vi "Prepare Elves - Unique Movement Order.vi"(1 "Movement Proposal Rules":T2(array[cluster]), 2 "Elves' Positions":bool[][](array[boolean])) -> (0 "Elves with Unique Movement Order":T3(c390))   [LabVIEW 2020, in "AoC 2022.lvlib"]
uses:
  AoC 2022.lvlib
  Day 15 - Beacon Exclusion Zone/private/Location.ctl
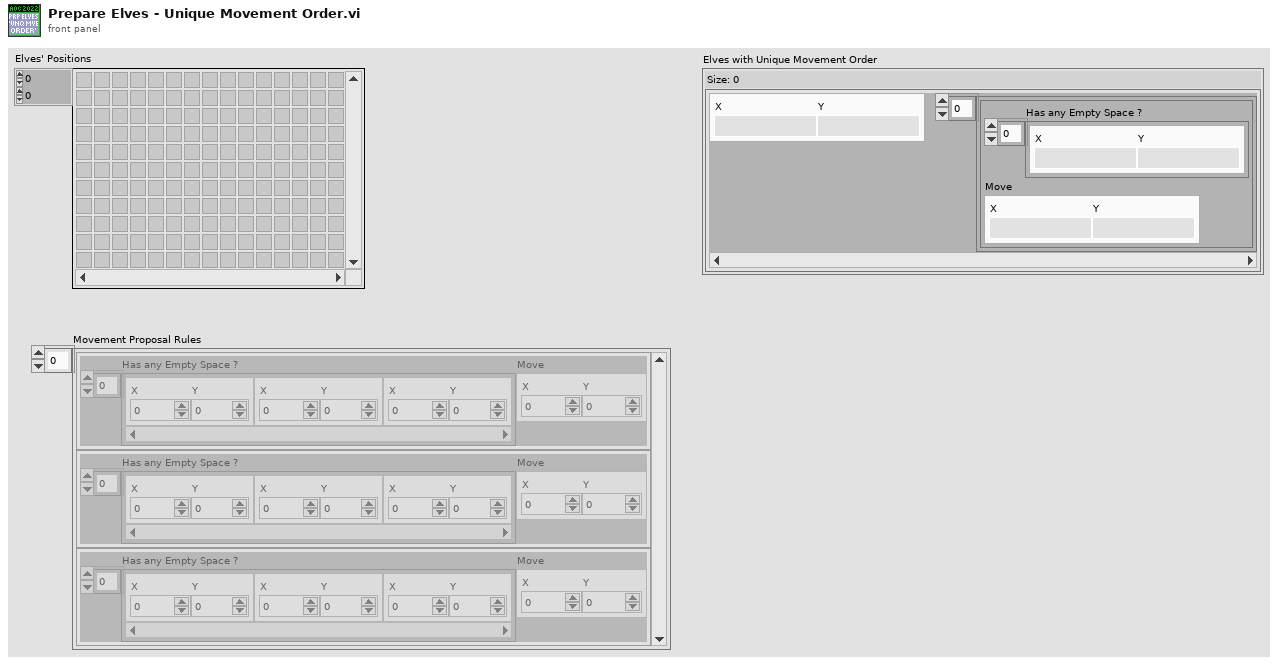
[diagram p1: front panel]
types:
  T1 = typedef "AoC 2022.lvlib/Location.ctl" = cluster{"X":i32, "Y":i32}
  T2 = cluster{"Has any Empty Space ?":T1[], "Move":T1}[]
  T3 = map{T1, cluster{"Has any Empty Space ?":T1[], "Move":T1}[]}
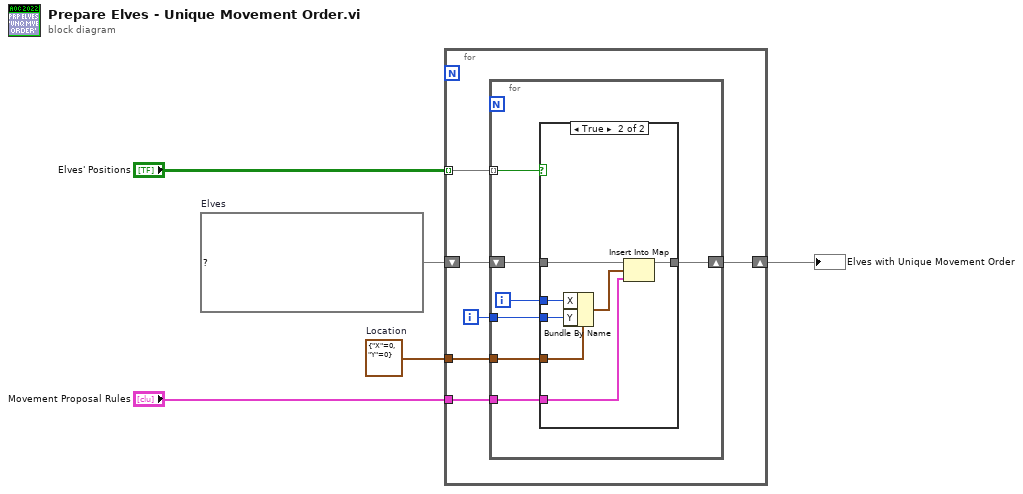
[diagram p0: block diagram]
diagram:
  w4 = T3 {}  # Elves
  w2 = T1 {"X"=0, "Y"=0}  # Location
  n1 = for {
    tunnel: "Elves' Positions" -> [w9] mode=indexing
    shift-right: [w11] -> w5
    shift-left: w4 -> [w10]
    tunnel: w2 -> [w8]
    tunnel: "Movement Proposal Rules" -> [w6]
    i -> [w7]
    n2 = for {
      shift-right: [w17] -> w11
      shift-left: w10 -> [w18]
      tunnel: w9 -> [w13] mode=indexing
      tunnel: w8 -> [w16]
      tunnel: w7 -> [w14]
      tunnel: w6 -> [w12]
      i -> [w15]
      n3 = case shown="True" w13 {
        tunnel: w18 -> [w19 w26]
        tunnel: [w19 w25] -> w17
        tunnel: w16 -> [_ w24]
        tunnel: w15 -> [_ w23]
        tunnel: w14 -> [_ w22]
        tunnel: w12 -> [_ w20]
        frame False {
        }
        frame True {
          n4 = Bundle By Name(cluster=w24, "X"=w23, "Y"=w22) -> (w21:T1)
          n5 = Insert Into Map(map in=w26, key=w21, value=w20) -> (map out=w25:T3)  [unwired: 2 out]
        }
      }
    }
  }
  "Elves with Unique Movement Order" <- w5
